vi "Tag Memory.vi"(5 "Tag In":T2, 7 "Tags":string[](array[string]), 8 "error in (no error)":errorcluster, 9 "Expected Type":T3, 10 "Tag":string, 11 "Method":T5) -> (0 "error out":errorcluster, 1 "Indices Out":i32[](array[numeric]), 2 "Description":string, 3 "Index Out":i32, 4 "Stored Tags":T1[](array[typedef]), 6 "Group Indices Out":T4[](array[typedef]))   [LabVIEW 2010, in "Current Value Table.lvlib"]
doc: "This VI stores the indices of every tag in the system, along with their type."
uses:
  Current Value Table.lvlib
  Tag Memory Methods.ctl
  Type Defs/Index Types.ctl
  Type Defs/Data Types.ctl
  Type Defs/Single Tag.ctl
  Type Defs/Tag in Memory.ctl
  ASCII String To Data.vi
  DataTypes/Double_ASCII String To Data.vi
  DataTypes/Array of String_ASCII String To Data.vi
  DataTypes/Array of Boolean_ASCII String To Data.vi
  DataTypes/Array of Single_ASCII String To Data.vi
  DataTypes/Array of Double_ASCII String To Data.vi
  DataTypes/Array of I8_ASCII String To Data.vi
  DataTypes/Array of I16_ASCII String To Data.vi
  DataTypes/Array of I32_ASCII String To Data.vi
  DataTypes/Array of I64_ASCII String To Data.vi
  DataTypes/Array of U64_ASCII String To Data.vi
  DataTypes/Array of U32_ASCII String To Data.vi
  DataTypes/Array of U16_ASCII String To Data.vi
  DataTypes/Array of U8_ASCII String To Data.vi
  DataTypes/Boolean_ASCII String To Data.vi
  DataTypes/String_ASCII String To Data.vi
  DataTypes/U8_ASCII String To Data.vi
  DataTypes/U16_ASCII String To Data.vi
  DataTypes/U32_ASCII String To Data.vi
  DataTypes/U64_ASCII String To Data.vi
  DataTypes/I8_ASCII String To Data.vi
  DataTypes/I16_ASCII String To Data.vi
  DataTypes/I32_ASCII String To Data.vi
  DataTypes/I64_ASCII String To Data.vi
  DataTypes/Single_ASCII String To Data.vi
  Errors/Scanned Value Error.vi
  Memory Block.vi
  DataTypes/Double_Memory Block.vi
  DataTypes/Array of String_Memory Block.vi
  DataTypes/Array of Boolean_Memory Block.vi
  DataTypes/Array of Single_Memory Block.vi
  DataTypes/Array of Double_Memory Block.vi
  DataTypes/Array of I8_Memory Block.vi
  DataTypes/Array of I16_Memory Block.vi
  DataTypes/Array of I32_Memory Block.vi
  DataTypes/Array of I64_Memory Block.vi
  DataTypes/Array of U64_Memory Block.vi
  DataTypes/Array of U32_Memory Block.vi
  DataTypes/Array of U16_Memory Block.vi
  DataTypes/Array of U8_Memory Block.vi
  DataTypes/Boolean_Memory Block.vi
  DataTypes/String_Memory Block.vi
  DataTypes/U8_Memory Block.vi
  DataTypes/U16_Memory Block.vi
  DataTypes/U32_Memory Block.vi
  DataTypes/U64_Memory Block.vi
  DataTypes/I8_Memory Block.vi
  DataTypes/I16_Memory Block.vi
  DataTypes/I32_Memory Block.vi
  DataTypes/I64_Memory Block.vi
  DataTypes/Single_Memory Block.vi
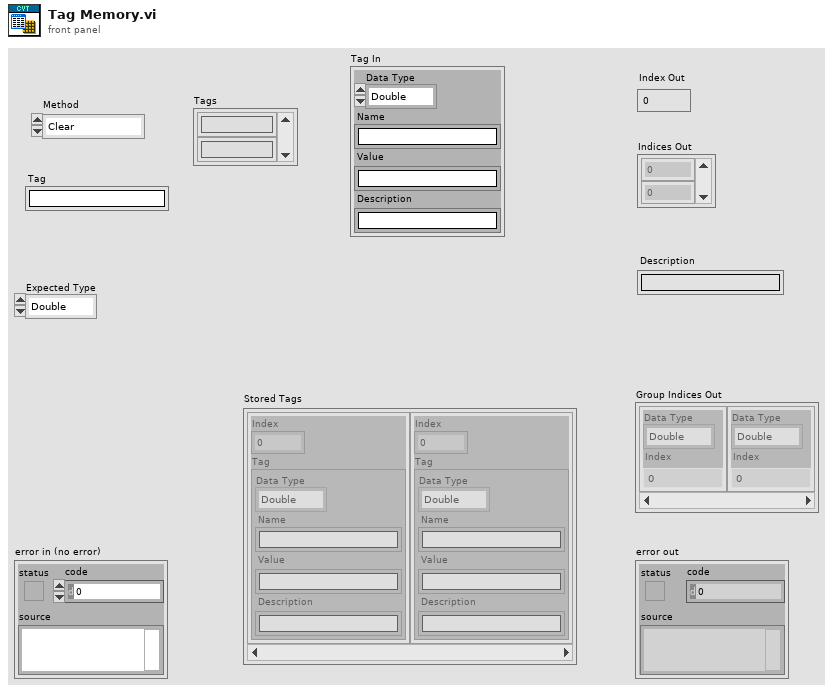
[diagram p1: front panel]
types:
  T1 = typedef "Current Value Table.lvlib/Tag in Memory.ctl" = cluster{"Index":i32, "Tag":T2}
  T2 = typedef "Current Value Table.lvlib/Single Tag.ctl" = cluster{"Data Type":T3, "Name":string, "Value":string, "Description":string}
  T3 = typedef "Current Value Table.lvlib/Data Types.ctl" = enum16{"Double", "Single", "I64", "I32", "I16", "I8", "U64", "U32", "U16", "U8", "String", "Boolean", "Array of U8", "Array of U16", "Array of U32", "Array of U64", "Array of I64", "Array of I32", "Array of I16", "Array of I8", "Array of Double", "Array of Single", "Array of Boolean", "Array of String"}
  T4 = typedef "Current Value Table.lvlib/Index Types.ctl" = cluster{"Data Type":T3, "Index":i32}
  T5 = typedef "Current Value Table.lvlib/Tag Memory Methods.ctl" = enum16{"Clear", "Read Tag Index", "Read Tag Indices", "Generate Group", "Add Tag", "Overwrite Tag", "Read Description", "Get Stored Tags"}
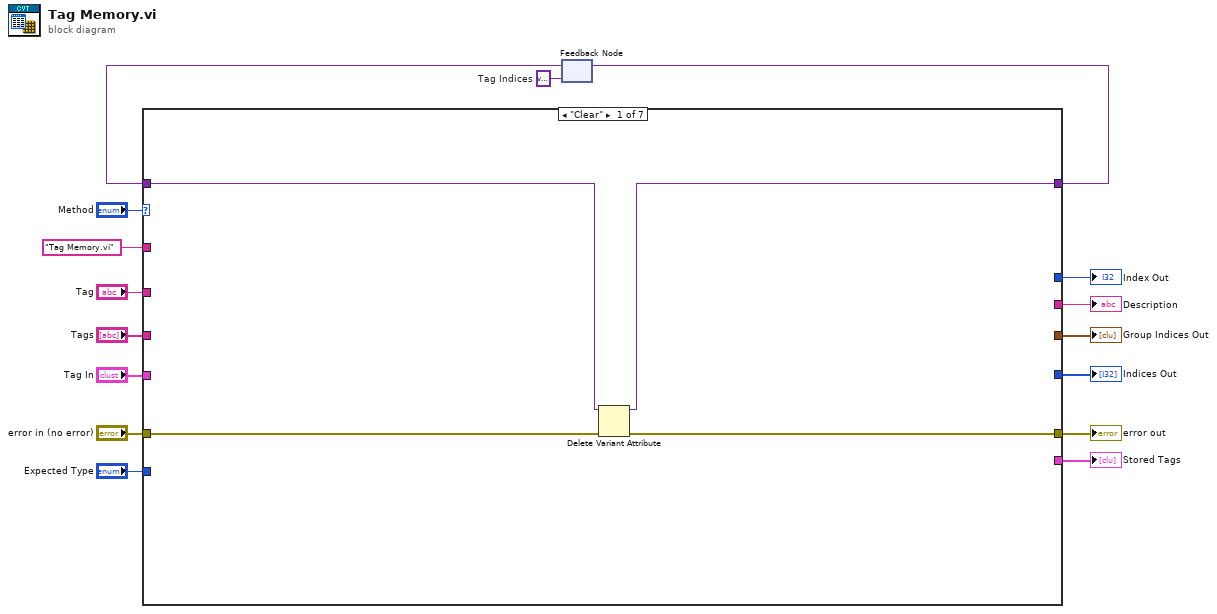
[diagram p0: block diagram]
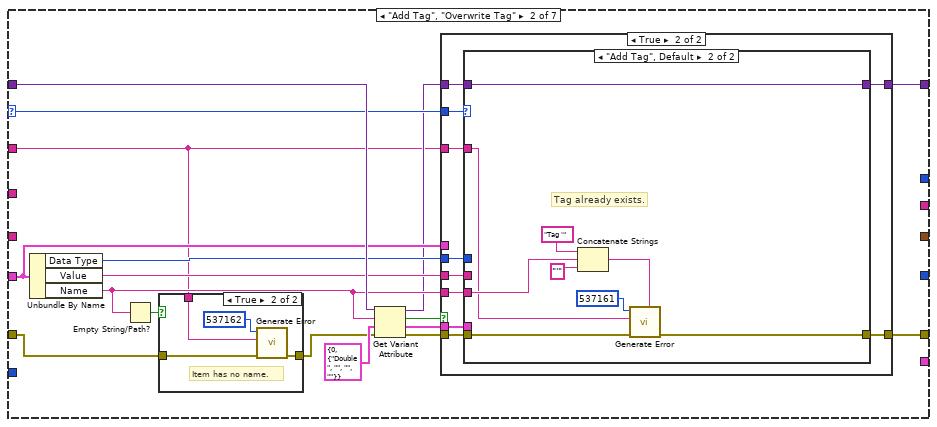
[diagram p2: hidden frame]
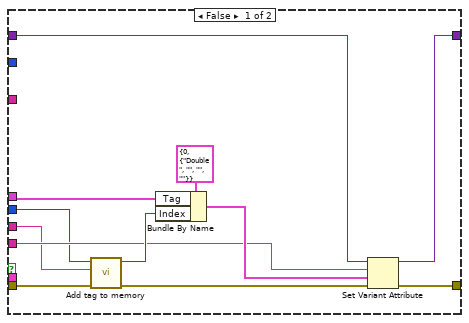
[diagram p4: hidden frame]
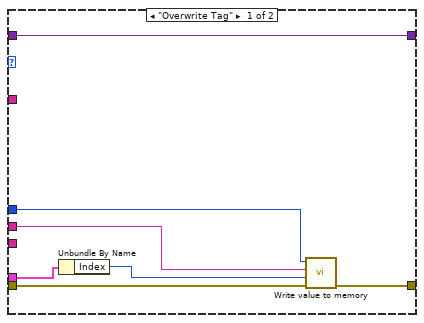
[diagram p5: hidden frame]
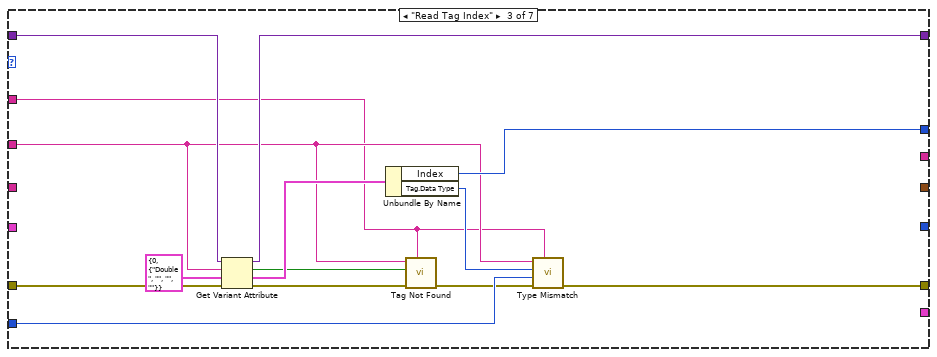
[diagram p6: hidden frame]
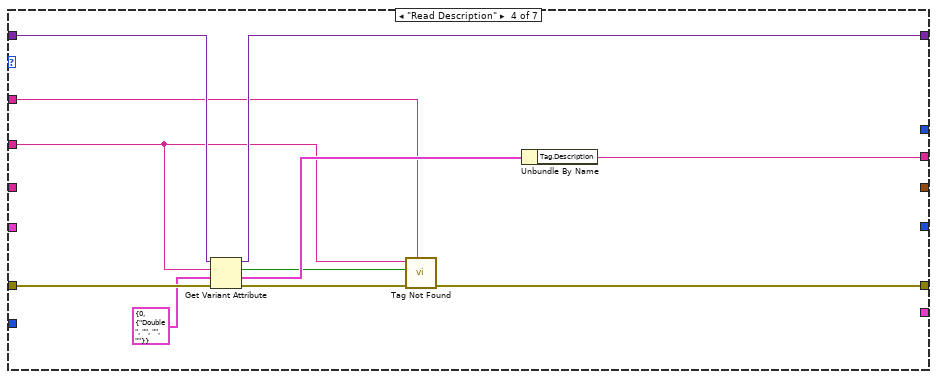
[diagram p7: hidden frame]
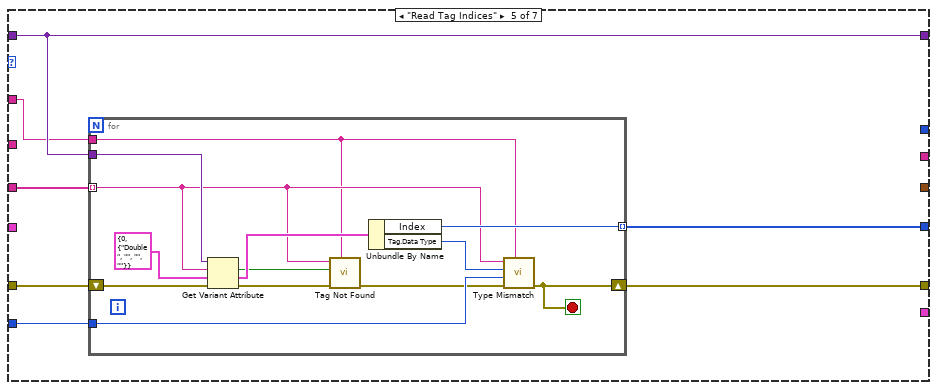
[diagram p8: hidden frame]
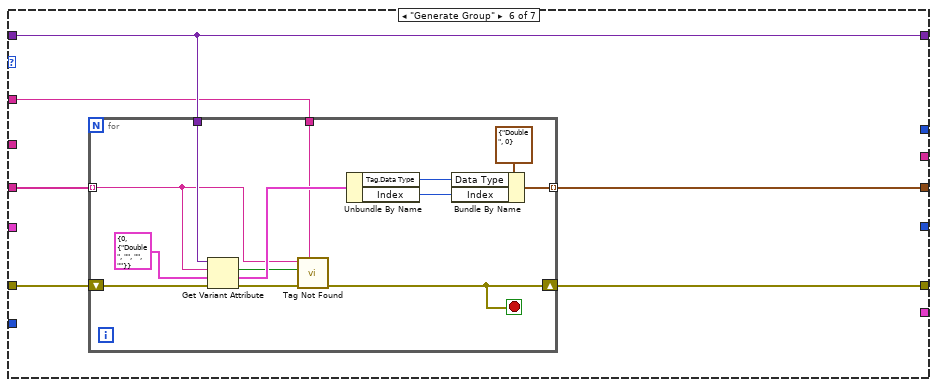
[diagram p9: hidden frame]
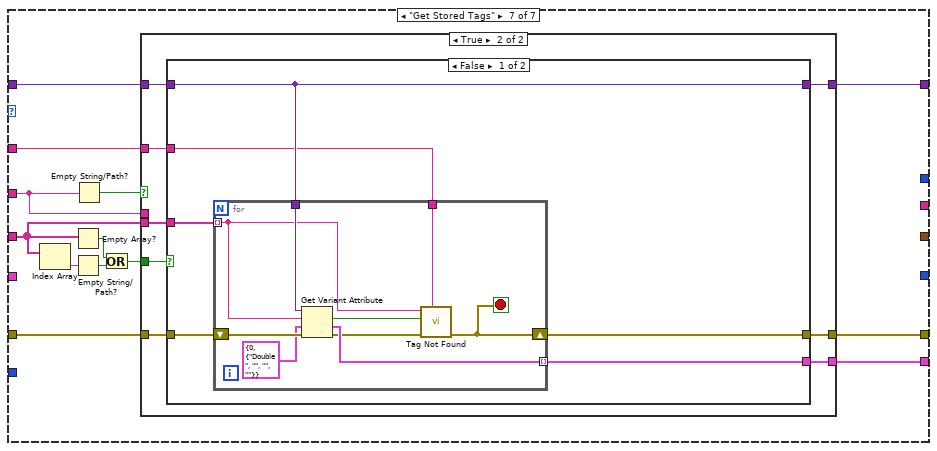
[diagram p10: hidden frame]
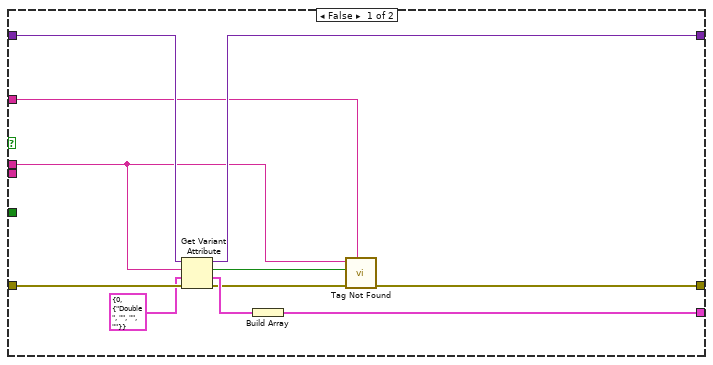
[diagram p11: hidden frame]
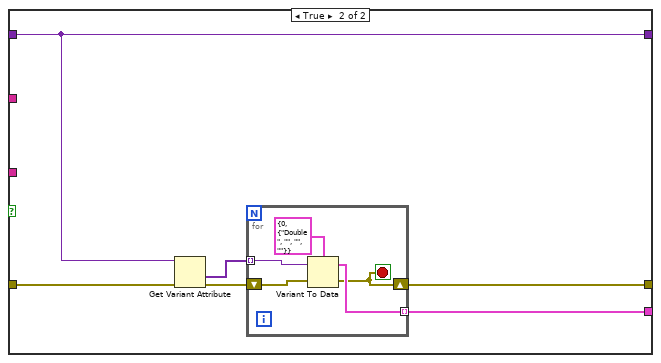
[diagram p12: hidden frame]
diagram:
  w16 = variant  # Tag Indices
  n1 = feedback #1(w16) -> (w14:variant)
  n2 = case shown="\"Clear\"" "Method" {
    selector: "Method" -> [_ w28 _ _ _ _ _]
    tunnel: w14 -> [w18 w37 w93 w104 w110 w129 w153]
    tunnel: [w17 w25 w92 w103 w110 w129 w152] -> w13
    tunnel: "Tag In" -> [_ w35 _ _ _ _ _]
    tunnel: "error in (no error)" -> [w20 w23 w94 w105 w112 w131 w155]
    tunnel: [w19 w26 w88 w98 w111 w130 w151] -> w10
    tunnel: "Tags" -> [_ _ _ _ w109 w128 w146]
    tunnel: [_ _ _ _ _ w127 _] -> w8
    tunnel: "Tag" -> [_ _ w83 w97 _ _ w154]
    tunnel: "Expected Type" -> [_ _ w86 _ w108 _ _]
    tunnel: [_ _ w89 _ _ _ _] -> w5
    tunnel: [_ _ _ w100 _ _ _] -> w4
    tunnel: [_ _ _ _ _ _ w150] -> w3
    tunnel: [_ _ _ _ w107 _ _] -> w2
    tunnel: "Tag Memory.vi" ("caller name") -> [_ w21 w81 w95 w106 w126 w145]
    frame "Clear" {
      n3 = Delete Variant Attribute(4:w20, 7:w18) -> (0:w19:errorcluster, 3:w17:variant)  [unwired: 1 in, 1 out]
    }
    frame "Add Tag", "Overwrite Tag" {
      n4 = Unbundle By Name(w35) -> ("Data Type"=w33:T3, "Value"=w32:string, "Name"=w34:string)
      n5 = Empty String/Path?(string/path=w34) -> (empty?=w24:bool)
      n6 = case shown="True" w24 {
        tunnel: w23 -> [w38 w41]
        tunnel: [w38 w40] -> w22
        tunnel: w21 -> [_ w39]
        frame False {
        }
        frame True {
          # "Item has no name."
          n7 = call "Generate Error.vi"("error in"=w41, "caller name"=w39, "code"=537162) -> ("error out"=w40:errorcluster)  [unwired: 8 in]
        }
      }
      n8 = Get Variant Attribute(Variant=w37, name=w34, default value (empty Variant)=T1 {"Index"=0, "Tag"={"Data Type"=enum."Double", "Name"="", "Value"="", "Description"=""}} ("Tag"), error in=w22) -> (duplicate Variant=w27:variant, found=w30:bool, value=w29:T1, error out=w36:errorcluster)
      n9 = case shown="True" w30 {
        tunnel: w36 -> [w49 w63]
        tunnel: w35 -> [w47 _]
        tunnel: w34 -> [w46 w60]
        tunnel: [w54 w62] -> w26
        tunnel: w33 -> [w44 w59]
        tunnel: w32 -> [w45 w58]
        tunnel: w29 -> [_ w61]
        tunnel: w28 -> [_ w64]
        tunnel: w27 -> [w53 w57]
        tunnel: [w52 w56] -> w25
        tunnel: w21 -> [_ w55]
        frame False {
          n10 = call "Add tag to memory.vi"("error in (no error)"=w49, "Value"=w45, "Data Type"=w44) -> ("error out"=w43:errorcluster, "Index"=w50:i32)  [unwired: 7 in]
          n11 = Bundle By Name(cluster=T1 {"Index"=0, "Tag"={"Data Type"=enum."Double", "Name"="", "Value"="", "Description"=""}} ("Tag"), "Tag"=w47, "Index"=w50) -> (w48:T1)
          n12 = Set Variant Attribute(Variant=w53, name=w46, value=w48, error in=w43) -> (Variant out=w52:variant, error out=w54:errorcluster)  [unwired: 1 out]
        }
        frame True {
          n13 = case shown="\"Add Tag\", Default" w64 {
            tunnel: w63 -> [w71 w74]
            tunnel: [w70 w73] -> w62
            tunnel: w61 -> [w66 _]
            tunnel: w60 -> [_ w76]
            tunnel: w59 -> [w69 _]
            tunnel: w58 -> [w68 _]
            tunnel: w57 -> [w65 w80]
            tunnel: [w65 w80] -> w56
            tunnel: w55 -> [_ w72]
            frame "Overwrite Tag" {
              n14 = Unbundle By Name(w66) -> ("Index"=w67:i32)
              n15 = call "Write value to memory.vi"("error in (no error)"=w71, "Index"=w67, "Value"=w68, "Data Type"=w69) -> ("error out"=w70:errorcluster)  [unwired: 7 in]
            }
            frame "Add Tag", Default {
              # "Tag already exists."
              n16 = Concatenate Strings("Tag '" ("string"), w76, "'" ("string")) -> (w75:string)
              n17 = call "Generate Error.vi"("<append> (\"\")"=w75, "error in"=w74, "caller name"=w72, "code"=537161) -> ("error out"=w73:errorcluster)  [unwired: 7 in]
            }
          }
        }
      }
    }
    frame "Read Tag Index" {
      n18 = Get Variant Attribute(Variant=w93, name=w83, default value (empty Variant)=T1 {"Index"=0, "Tag"={"Data Type"=enum."Double", "Name"="", "Value"="", "Description"=""}} ("Tag"), error in=w94) -> (duplicate Variant=w92:variant, found=w82:bool, value=w90:T1, error out=w85:errorcluster)
      n19 = Unbundle By Name(w90) -> ("Index"=w89:i32, "Tag.Data Type"=w87:T3)
      n20 = call "Tag Not Found.vi"("caller name"=w81, "error in (no error)"=w85, "found?"=w82, "Tag Name"=w83) -> ("error out"=w84:errorcluster)  [unwired: 7 in]
      n21 = call "Type Mismatch.vi"("caller name"=w81, "error in (no error)"=w84, "Data Type Requested"=w86, "True Type"=w87, "Tag"=w83) -> ("error out"=w88:errorcluster)  [unwired: 6 in]
    }
    frame "Read Description" {
      n22 = Get Variant Attribute(Variant=w104, name=w97, default value (empty Variant)=T1 {"Index"=0, "Tag"={"Data Type"=enum."Double", "Name"="", "Value"="", "Description"=""}} ("Tag"), error in=w105) -> (duplicate Variant=w103:variant, found=w96:bool, value=w101:T1, error out=w99:errorcluster)
      n23 = call "Tag Not Found.vi"("caller name"=w95, "error in (no error)"=w99, "found?"=w96, "Tag Name"=w97) -> ("error out"=w98:errorcluster)  [unwired: 7 in]
      n24 = Unbundle By Name(w101) -> ("Tag.Description"=w100:string)
    }
    frame "Read Tag Indices" {
      n25 = for {
        shift-right: [w121] -> w111
        shift-left: w112 -> [w125]
        tunnel: w110 -> [w123]
        tunnel: w109 -> [w117] mode=indexing
        tunnel: w108 -> [w120]
        tunnel: [w118] -> w107 mode=indexing
        tunnel: w106 -> [w113]
        stop <- w121 stop-if-true
        n26 = Get Variant Attribute(Variant=w123, name=w117, default value (empty Variant)=T1 {"Index"=0, "Tag"={"Data Type"=enum."Double", "Name"="", "Value"="", "Description"=""}} ("Tag"), error in=w125) -> (found=w116:bool, value=w122:T1, error out=w115:errorcluster)  [unwired: 1 out]
        n27 = call "Tag Not Found.vi"("caller name"=w113, "error in (no error)"=w115, "found?"=w116, "Tag Name"=w117) -> ("error out"=w114:errorcluster)  [unwired: 7 in]
        n28 = Unbundle By Name(w122) -> ("Index"=w118:i32, "Tag.Data Type"=w119:T3)
        n29 = call "Type Mismatch.vi"("caller name"=w113, "error in (no error)"=w114, "Data Type Requested"=w120, "True Type"=w119, "Tag"=w117) -> ("error out"=w121:errorcluster)  [unwired: 6 in]
      }
    }
    frame "Generate Group" {
      n30 = for {
        shift-right: [w135] -> w130
        shift-left: w131 -> [w144]
        tunnel: w129 -> [w142]
        tunnel: w128 -> [w133] mode=indexing
        tunnel: [w140] -> w127 mode=indexing
        tunnel: w126 -> [w132]
        stop <- w135 stop-if-true
        n31 = Get Variant Attribute(Variant=w142, name=w133, default value (empty Variant)=T1 {"Index"=0, "Tag"={"Data Type"=enum."Double", "Name"="", "Value"="", "Description"=""}} ("Tag"), error in=w144) -> (found=w134:bool, value=w139:T1, error out=w136:errorcluster)  [unwired: 1 out]
        n32 = call "Tag Not Found.vi"("caller name"=w132, "error in (no error)"=w136, "found?"=w134, "Tag Name"=w133) -> ("error out"=w135:errorcluster)  [unwired: 7 in]
        n33 = Unbundle By Name(w139) -> ("Tag.Data Type"=w137:T3, "Index"=w138:i32)
        n34 = Bundle By Name(cluster=T4 {"Data Type"=enum."Double", "Index"=0} ("Index Type"), "Data Type"=w137, "Index"=w138) -> (w140:T4)
      }
    }
    frame "Get Stored Tags" {
      n35 = Index Array(array=w146) -> (element=w157:string)  [unwired: 1 in]
      n36 = Empty Array?(array=w146) -> (empty?=w148:bool)
      n37 = Empty String/Path?(string/path=w157) -> (empty?=w149:bool)
      n38 = Empty String/Path?(string/path=w154) -> (empty?=w156:bool)
      n39 = Or(x=w148, y=w149) -> (x .or. y?=w147:bool)
      n40 = case shown="True" w156 {
        tunnel: w155 -> [w168 w176]
        tunnel: w154 -> [w159 _]
        tunnel: w153 -> [w167 w173]
        tunnel: [w166 w172] -> w152
        tunnel: [w161 w175] -> w151
        tunnel: [w163 w171] -> w150
        tunnel: w147 -> [_ w174]
        tunnel: w146 -> [_ w170]
        tunnel: w145 -> [w158 w169]
        frame False {
          n41 = Get Variant Attribute(Variant=w167, name=w159, default value (empty Variant)=T1 {"Index"=0, "Tag"={"Data Type"=enum."Double", "Name"="", "Value"="", "Description"=""}} ("Tag"), error in=w168) -> (duplicate Variant=w166:variant, found=w160:bool, value=w164:T1, error out=w162:errorcluster)
          n42 = Build Array(w164) -> (w163:T1[])
          n43 = call "Tag Not Found.vi"("caller name"=w158, "error in (no error)"=w162, "found?"=w160, "Tag Name"=w159) -> ("error out"=w161:errorcluster)  [unwired: 7 in]
        }
        frame True {
          n44 = case shown="False" w174 {
            tunnel: w176 -> [w182 w197]
            tunnel: [w181 w194] -> w175
            tunnel: w173 -> [w179 w196]
            tunnel: [w179 w196] -> w172
            tunnel: [w178 w192] -> w171
            tunnel: w170 -> [w180 _]
            tunnel: w169 -> [w177 _]
            frame False {
              n45 = for {
                shift-right: [w186] -> w181
                shift-left: w182 -> [w191]
                tunnel: w180 -> [w184] mode=indexing
                tunnel: w179 -> [w189]
                tunnel: [w188] -> w178 mode=indexing
                tunnel: w177 -> [w183]
                stop <- w186 stop-if-true
                n46 = Get Variant Attribute(Variant=w189, name=w184, default value (empty Variant)=T1 {"Index"=0, "Tag"={"Data Type"=enum."Double", "Name"="", "Value"="", "Description"=""}} ("Tag"), error in=w191) -> (found=w185:bool, value=w188:T1, error out=w187:errorcluster)  [unwired: 1 out]
                n47 = call "Tag Not Found.vi"("caller name"=w183, "error in (no error)"=w187, "found?"=w185, "Tag Name"=w184) -> ("error out"=w186:errorcluster)  [unwired: 7 in]
              }
            }
            frame True {
              n48 = Get Variant Attribute(Variant=w196, error in=w197) -> (values=w193:variant[], error out=w195:errorcluster)  [unwired: 2 in, 2 out]
              n49 = for {
                shift-right: [w198] -> w194
                shift-left: w195 -> [w202]
                tunnel: w193 -> [w200] mode=indexing
                tunnel: [w199] -> w192 mode=indexing
                stop <- w198 stop-if-true
                n50 = Variant To Data(error in=w202, Variant=w200, type=T1 {"Index"=0, "Tag"={"Data Type"=enum."Double", "Name"="", "Value"="", "Description"=""}} ("Tag")) -> (error out=w198:errorcluster, data=w199:T1)
              }
            }
          }
        }
      }
    }
  }
  "error out" <- w10
  "Group Indices Out" <- w8
  "Index Out" <- w5
  "Description" <- w4
  "Stored Tags" <- w3
  "Indices Out" <- w2
  n51 = feedback-in #1(w13) -> ()
